vi "Condition Retrieve Record.vi"(8 "error in (no error)":errorcluster, 11 "Statement Refnum":T1) -> (0 "error out":errorcluster, 2 "Condition":T2, 3 "Statement Refnum":T1)   [LabVIEW 2011]
uses:
  Condition Record.ctl
  Condition Operators.ctl
  Summitek EXT/ODBC/SQL Controls/Statement Refnum.ctl
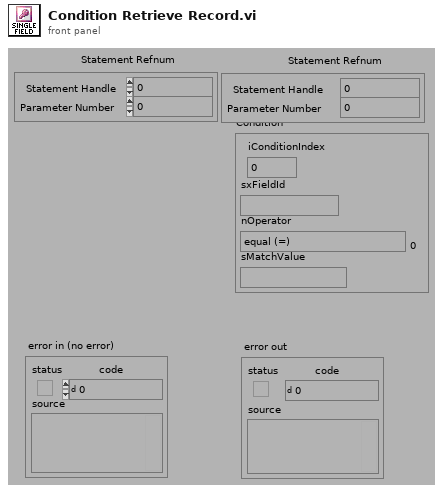
[diagram p1: front panel]
types:
  T1 = typedef "Statement Refnum.ctl" = cluster{"Statement Handle":i32, "Parameter Number":u16}
  T2 = typedef "Condition Record.ctl" = cluster{"iConditionIndex":i32, "sxFieldId":string, "nOperator":T3, "sMatchValue":string}
  T3 = typedef "Condition Operators.ctl" = enum16{"equal (=)", "not equal (\\u2260)", "less than (<)", "less than or equal (\\u2264)", "greater than (>)", "greater than or equal (\\u2265)", "contains", "does not contain"}
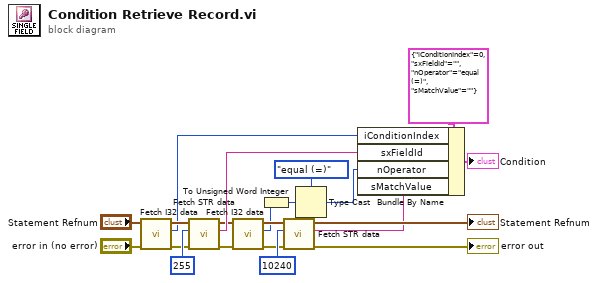
[diagram p0: block diagram]
diagram:
  n1 = call "Fetch I32 data.vi"("error in (no error)"="error in (no error)", "Statement Refnum"="Statement Refnum") -> ("error out"=w6:errorcluster, "Data"=w3:i32, "Statement Refnum"=w4:T1)  [unwired: 3 out]
  n2 = call "Fetch STR data.vi"("error in (no error)"=w6, "Buffer Size"=255, "Statement Refnum"=w4) -> ("error out"=w9:errorcluster, "Data"=w13:string, "Statement Refnum"=w11:T1)  [unwired: 2 out]
  n3 = call "Fetch I32 data.vi"("error in (no error)"=w9, "Statement Refnum"=w11) -> ("error out"=w8:errorcluster, "Data"=w2:i32, "Statement Refnum"=w10:T1)  [unwired: 3 out]
  n4 = To Unsigned Word Integer(number=w2) -> (unsigned 16bit integer=w1:u16)
  n5 = call "Fetch STR data.vi"("error in (no error)"=w8, "Buffer Size"=10240, "Statement Refnum"=w10) -> ("error out"=→"error out":errorcluster, "Data"=w12:string, "Statement Refnum"=→"Statement Refnum":T1)  [unwired: 2 out]
  n6 = Type Cast(type=Condition_Operators."equal (=)" ("nOperator"), x=w1) -> (*(type *) &x=w14:T3)
  n7 = Bundle By Name(cluster=T2 {"iConditionIndex"=0, "sxFieldId"="", "nOperator"=enum."equal (=)", "sMatchValue"=""} ("Field Data Information"), "iConditionIndex"=w3, "sxFieldId"=w13, "nOperator"=w14, "sMatchValue"=w12) -> (→"Condition":T2)
